vi "Read configuration.vi"(8 "error in (no error)":errorcluster, 11 "HiPOT Instrument in":refnum<class "HiPOT Instrument.lvclass">) -> (0 "error out":errorcluster, 2 "configuration":refnum<class "CEF_serializable configuration.lvclass">, 3 "HiPOT Instrument out":refnum<class "HiPOT Instrument.lvclass">)   [LabVIEW 2025, in "HiPOT.lvlib" / "HiPOT Instrument.lvclass"]
uses:
  HiPOT Instrument.lvclass
  Users/Public/Documents/Sandia National Labs/TSS Plugin/CEF.lvlibp/serializable configuration/CEF_serializable configuration.lvclass
  HiPOT Instrument.lvclass/HiPOT Instrument.ctl
  HiPOT configuration/HiPOT configuration.lvclass
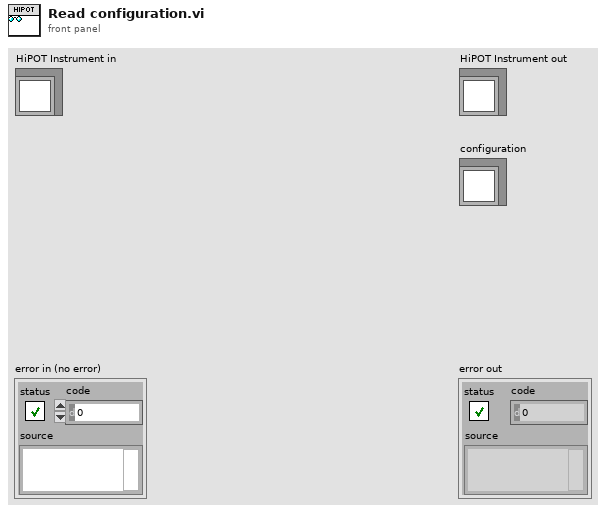
[diagram p1: front panel]
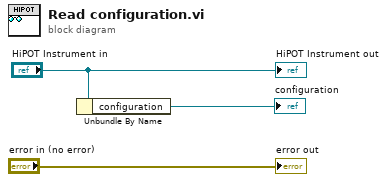
[diagram p0: block diagram]
diagram:
  n1 = Unbundle By Name("HiPOT Instrument in") -> ("configuration"=→"configuration":refnum<class "HiPOT configuration.lvclass">)
  "error out" <- "error in (no error)"
  "HiPOT Instrument out" <- "HiPOT Instrument in"
